vi "Enumerate Devices.vi"(8 "error in (no error)":errorcluster) -> (0 "error out":errorcluster, 3 "Devices":T1[](array[typedef]))   [LabVIEW 2020]
uses:
  Device Enumeration.ctl
  bin/gindustrialcam_32-1.dll
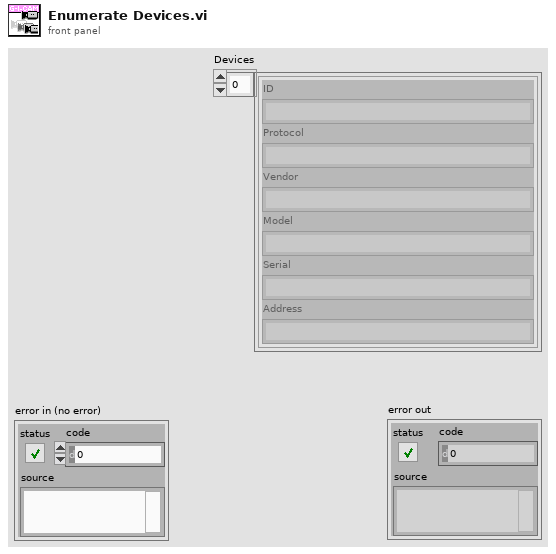
[diagram p1: front panel]
types:
  T1 = typedef "Device Enumeration.ctl" = cluster{"ID":string, "Protocol":string, "Vendor":string, "Model":string, "Serial":string, "Address":string}
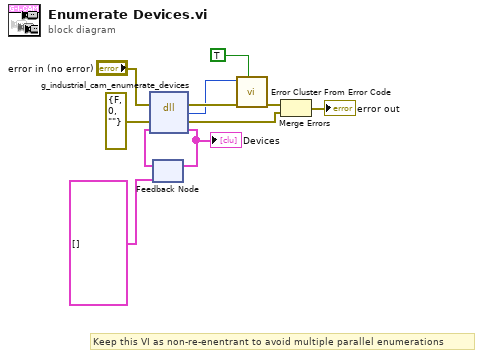
[diagram p0: block diagram]
diagram:
  # "Keep this VI as non-re-enentrant to avoid multiple parallel enumerations"
  n1 = feedback #1(T1[] [] ("Array")) -> (w1:T1[])
  n2 = dll-call lib="C:/Workspace/SSDC/g-industrial-camera/LabVIEW/g_industrial_cam/bin/gindustrialcam_*-1.*" fn="g_industrial_cam_enumerate_devices"(error in="error in (no error)", "Error"=errorcluster {"status"=FALSE, "code"=0, "source"=""} ("error constant"), "Enumeration"=w1) -> (error out=w9:errorcluster, "MgError"=w8:i32, "Error"=w5:errorcluster, "Enumeration"=w3:T1[])  [unwired: 2 in, 1 out]
  "Devices" <- w3
  n3 = feedback-in #1(w3) -> ()
  n4 = call <vilib>:"Error Cluster From Error Code.vi"("show call chain? (False)"=TRUE, "error in (no error)"=w9, "error code (0)"=w8) -> ("error out"=w6:errorcluster)  [unwired: 6 in]
  n5 = Merge Errors(w6, w5) -> (→"error out":errorcluster)
